vi "_digital_off.vi"(11 "digital port":tag="Dev1/port1/line2") -> ()   [LabVIEW 2024]
uses:
  <vilib>/DAQmx/write.llb/DAQmx Write (Digital Bool 1Line 1Point).vi
  <vilib>/DAQmx/create/channels.llb/DAQmx Create Channel (DO-Digital Output).vi
  <vilib>/DAQmx/miscellaneous.llb/DAQmx Fill In Error Info.vi
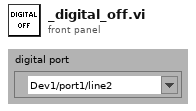
[diagram p1: front panel]
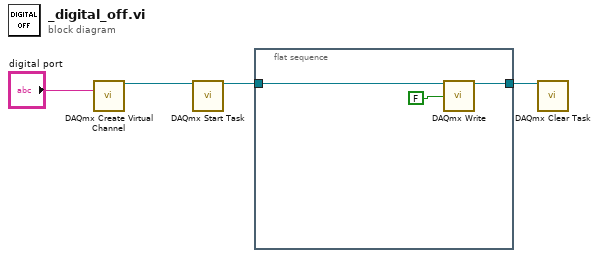
[diagram p0: block diagram]
diagram:
  n1 = call-poly <vilib>:"DAQmx Create Virtual Channel.vi"("lines"="digital port") -> ("task out"=w3:refnum<k21>)  [unwired: 13 in, 1 out]
  n2 = call <vilib>:"DAQmx Start Task.vi"("task/channels in"=w3) -> ("task out"=w2:refnum<k21>)  [unwired: 13 in, 1 out]
  n3 = flat-sequence {
    tunnel: [w6] -> w1
    tunnel: w2 -> [w7]
    frame #0 {
      n4 = call-poly <vilib>:"DAQmx Write.vi"("task/channels in"=w7, "data"=FALSE) -> ("task out"=w6:refnum<k21>)  [unwired: 11 in, 2 out]
    }
  }
  n5 = call <vilib>:"DAQmx Clear Task.vi"("task in"=w1) -> ()  [unwired: 14 in, 1 out]
